vi "Read Write Last Configured Value.vi"(0 "Template Sequence Path":path=path "C:/Projects/STS/QPA88xx/QPA88XX Template 2p3.seq", 1 "Use Existing Test Numbers?":bool, 5 "New Sequence File Path":path=path "C:/Projects/STS/QPA88xx/EN4N-P512X-1AAA.seq", 7 "Test Conditions File":path=path "C:/Users/c_arumu/Desktop/QPA88xx_TCF_rev012.xlsx", 9 "Limits File Path":path=path "C:/Projects/STS/QPA88xx/TestLimits/CalcLimits_EN1N-P512X-12A - Copy.txt", 11 "error in (no error)":errorcluster, 12 "Create Focus Calibration Definition File?":bool=TRUE, 13 "Write?":bool) -> (3 "Use Existing Test Numbers? 2":bool, 4 "Template Sequence":path, 6 "New Sequence File":path, 8 "Test Conditions File":path, 10 "Limits File":path, 14 "Create Focus Calibration Definition File? 2":bool=TRUE, 15 "error out":errorcluster)   [LabVIEW 2018]
uses:
  <vilib>/Utility/config.llb/Write Key (Path).vi
  <vilib>/Utility/config.llb/Write Key (Boolean).vi
  <vilib>/Utility/config.llb/Read Key (Path).vi
  <vilib>/Utility/config.llb/Read Key (Boolean).vi
  <vilib>/Utility/config.llb/NI_LVConfig.lvlib
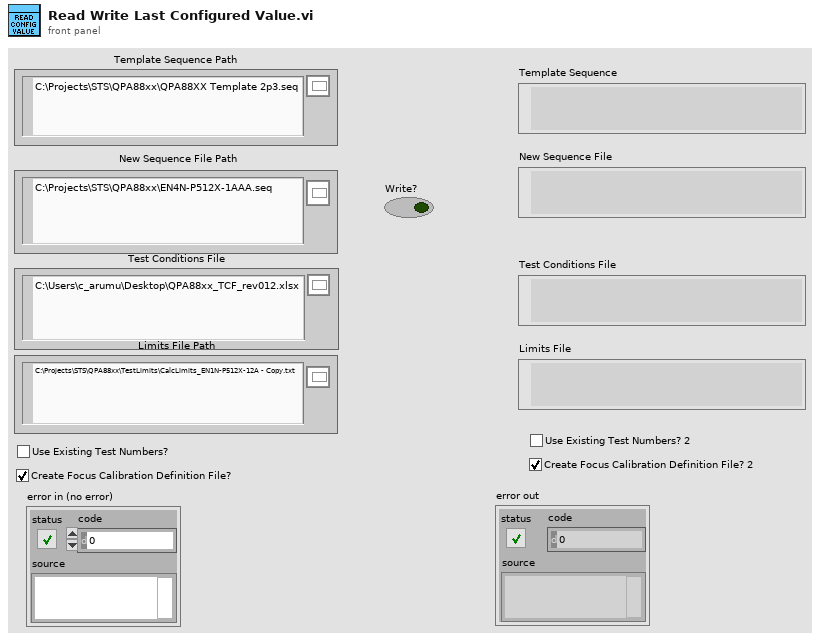
[diagram p1: front panel]
types:
  T1 = enum32{"invalid app kind", "Development System", "Run Time System", "Student Edition", "Embedded LabVIEW", "Evaluation", "Custom"}
  T2 = typedef "NI_LVConfig.lvlib/Config Data RefNum.ctl" = refnum<k1>
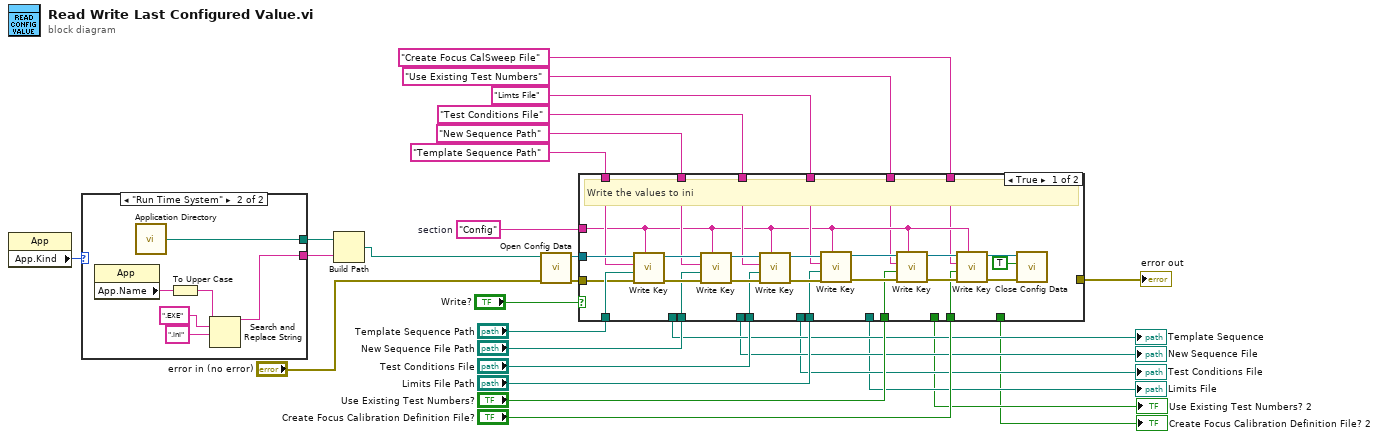
[diagram p0: block diagram]
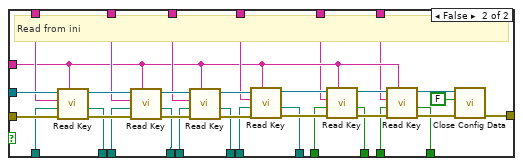
[diagram p2: hidden frame]
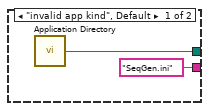
[diagram p3: hidden frame]
diagram:
  w15 = "Config"  # section
  n1 = property class="App"() -> ("App.Kind"=w28:T1)  [unwired: 2 in, 2 out]
  n2 = case shown="\"Run Time System\"" w28 {
    tunnel: [w30 w36] -> w27
    tunnel: ["SeqGen.ini" w31] -> w26
    frame "invalid app kind", Default {
      n3 = call <vilib>:"Application Directory.vi"() -> ("Application Directory"=w30:path)
    }
    frame "Run Time System" {
      n4 = property class="App"() -> ("App.Name"=w33:string)  [unwired: 2 in, 2 out]
      n5 = call <vilib>:"Application Directory.vi"() -> ("Application Directory"=w36:path)
      n6 = To Upper Case(1:w33) -> (0:w32:string)
      n7 = Search and Replace String(input string=w32, search string=".EXE" ("substring (\"\")"), replace string=".ini" ("replace string (\"\")")) -> (result string=w31:string)  [unwired: 5 in, 3 out]
    }
  }
  n8 = Build Path(base path=w27, name or relative path=w26) -> (appended path=w10:path)
  n9 = call <vilib>:"Open Config Data.vi"("error in (no error)"="error in (no error)", "configuration file path"=w10) -> ("error out"=w22:errorcluster, "refnum"=w25:T2)  [unwired: 7 in, 1 out]
  n10 = case shown="True" "Write?" {
    tunnel: w25 -> [w64 w99]
    tunnel: "Template Sequence Path" ("key") -> [w63 w98]
    tunnel: "Template Sequence Path" -> [w62 w73]
    tunnel: w22 -> [w61 w97]
    tunnel: "New Sequence Path" ("key") -> [w58 w94]
    tunnel: "New Sequence File Path" -> [w57 w76]
    tunnel: "Test Conditions File" ("key") -> [w54 w91]
    tunnel: "Test Conditions File" -> [w53 w75]
    tunnel: "Limts File" ("key") -> [w50 w88]
    tunnel: "Limits File Path" -> [w49 w74]
    tunnel: w15 -> [w44 w83]
    tunnel: "Use Existing Test Numbers" ("key") -> [w43 w82]
    tunnel: "Create Focus CalSweep File" ("key") -> [w42 w81]
    tunnel: "Use Existing Test Numbers?" -> [w41 w80]
    tunnel: "Create Focus Calibration Definition File?" -> [w40 w79]
    tunnel: [_ w71] -> w8
    tunnel: [_ w70] -> w7
    tunnel: [_ w69] -> w6
    tunnel: [_ w68] -> w5
    tunnel: [_ w67] -> w4
    tunnel: [_ w66] -> w3
    tunnel: [_ w65] -> w2
    frame True {
      # "Write the values to ini"
      n11 = call-poly <vilib>:"Write Key.vi"("section"=w44, "error in (no error)"=w61, "value"=w62, "key"=w63, "refnum"=w64) -> ("error out"=w60:errorcluster, "refnum out"=w59:T2)  [unwired: 4 in, 1 out]
      n12 = call-poly <vilib>:"Write Key.vi"("section"=w44, "error in (no error)"=w60, "value"=w57, "key"=w58, "refnum"=w59) -> ("error out"=w56:errorcluster, "refnum out"=w55:T2)  [unwired: 4 in, 1 out]
      n13 = call-poly <vilib>:"Write Key.vi"("section"=w44, "error in (no error)"=w56, "value"=w53, "key"=w54, "refnum"=w55) -> ("error out"=w52:errorcluster, "refnum out"=w51:T2)  [unwired: 4 in, 1 out]
      n14 = call-poly <vilib>:"Write Key.vi"("section"=w44, "error in (no error)"=w52, "value"=w49, "key"=w50, "refnum"=w51) -> ("error out"=w48:errorcluster, "refnum out"=w47:T2)  [unwired: 4 in, 1 out]
      n15 = call-poly <vilib>:"Write Key.vi"("section"=w44, "error in (no error)"=w48, "value"=w41, "key"=w43, "refnum"=w47) -> ("error out"=w46:errorcluster, "refnum out"=w45:T2)  [unwired: 4 in, 1 out]
      n16 = call-poly <vilib>:"Write Key.vi"("section"=w44, "error in (no error)"=w46, "value"=w40, "key"=w42, "refnum"=w45) -> ("error out"=w38:errorcluster, "refnum out"=w39:T2)  [unwired: 4 in, 1 out]
      n17 = call <vilib>:"Close Config Data.vi"("error in (no error)"=w38, "write file if changed (T)"=TRUE, "refnum"=w39) -> ()  [unwired: 7 in, 2 out]
    }
    frame False {
      # "Read from ini"
      n18 = call-poly <vilib>:"Read Key.vi"("section"=w83, "error in (no error)"=w97, "default value"=w73, "key"=w98, "refnum"=w99) -> ("error out"=w96:errorcluster, "value"=w71:path, "refnum out"=w95:T2)  [unwired: 3 in, 1 out]
      n19 = call-poly <vilib>:"Read Key.vi"("section"=w83, "error in (no error)"=w96, "default value"=w76, "key"=w94, "refnum"=w95) -> ("error out"=w93:errorcluster, "value"=w70:path, "refnum out"=w92:T2)  [unwired: 3 in, 1 out]
      n20 = call-poly <vilib>:"Read Key.vi"("section"=w83, "error in (no error)"=w93, "default value"=w75, "key"=w91, "refnum"=w92) -> ("error out"=w90:errorcluster, "value"=w69:path, "refnum out"=w89:T2)  [unwired: 3 in, 1 out]
      n21 = call-poly <vilib>:"Read Key.vi"("section"=w83, "error in (no error)"=w90, "default value"=w74, "key"=w88, "refnum"=w89) -> ("error out"=w87:errorcluster, "value"=w68:path, "refnum out"=w86:T2)  [unwired: 3 in, 1 out]
      n22 = call-poly <vilib>:"Read Key.vi"("section"=w83, "error in (no error)"=w87, "default value"=w80, "key"=w82, "refnum"=w86) -> ("error out"=w85:errorcluster, "value"=w67:bool, "refnum out"=w84:T2)  [unwired: 3 in, 1 out]
      n23 = call-poly <vilib>:"Read Key.vi"("section"=w83, "error in (no error)"=w85, "default value"=w79, "key"=w81, "refnum"=w84) -> ("error out"=w77:errorcluster, "value"=w66:bool, "refnum out"=w78:T2)  [unwired: 3 in, 1 out]
      n24 = call <vilib>:"Close Config Data.vi"("error in (no error)"=w77, "write file if changed (T)"=FALSE, "refnum"=w78) -> ("error out"=w65:errorcluster)  [unwired: 7 in, 1 out]
    }
  }
  "Template Sequence" <- w8
  "New Sequence File" <- w7
  "Test Conditions File" <- w6
  "Limits File" <- w5
  "Use Existing Test Numbers? 2" <- w4
  "Create Focus Calibration Definition File? 2" <- w3
  "error out" <- w2
